vi "P4CMD Configure Project.vi"(8 "error in (no error)":errorcluster, 9 "configuration data in":string) -> (0 "error out":errorcluster, 1 "configuration data out":string, 2 "status message":string, 5 "dialog box cancelled?":bool)   [LabVIEW 2020, in "NI_SCC_P4CMD.lvlib"]
uses:
  <vilib>/SourceControl/Providers/P4CMD/NI_SCC_P4CMD.lvlib
  <vilib>/SourceControl/support/SCCSup Message Strings GLBL.vi
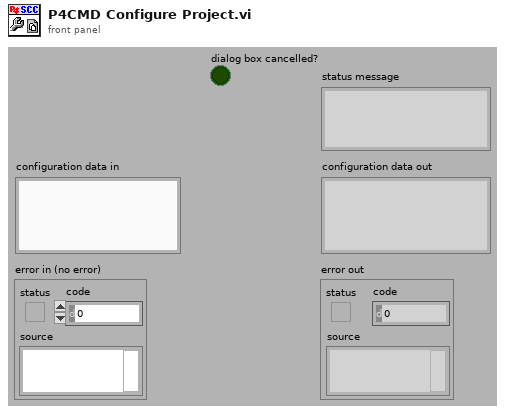
[diagram p1: front panel]
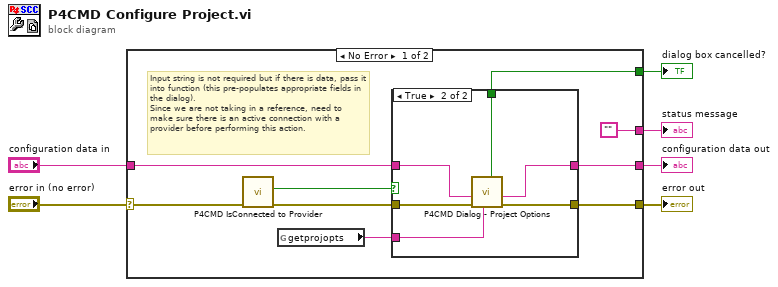
[diagram p0: block diagram]
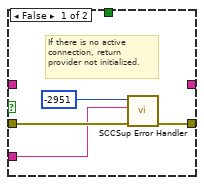
[diagram p2: hidden frame]
diagram:
  n1 = case shown="No Error" "error in (no error)" {
    selector: "error in (no error)" -> [w11 w26]
    tunnel: [w8 w26] -> w5
    tunnel: ["" _] -> w4
    tunnel: [w12 _] -> w3
    tunnel: [w13 _] -> w2
    tunnel: "configuration data in" -> [w14 _]
    frame No Error {
      # "Input string is not required but if there is data, pass it into function (this pre-populates appropriate fields in the dialog).\nSince we are not taking in a reference, need to make sure there is an active connection with a provider before performing this action."
      n2 = call <vilib>:"P4CMD IsConnected to Provider.vi"("error in (no error)"=w11) -> ("error out"=w10:errorcluster, "active connection?"=w9:bool)  [unwired: 9 in]
      n3 = global read "SCCSup Message Strings GLBL.vi" "getprojopts"() -> (w7:string)
      n4 = case shown="True" w9 {
        tunnel: w14 -> [_ w25]
        tunnel: [w18 w24] -> w8
        tunnel: [_ w23] -> w13
        tunnel: [_ w22] -> w12
        tunnel: w10 -> [w19 w21]
        tunnel: w7 -> [w16 w20]
        frame False {
          # "If there is no active connection, return provider not initialized."
          n5 = call <vilib>:"SCCSup Error Handler.vi"("error in (no error)"=w19, "operation message"=w16, "scc error code"=-2951 ("t")) -> ("error out"=w18:errorcluster)  [unwired: 8 in]
        }
        frame True {
          n6 = call <vilib>:"P4CMD Dialog - Project Options.vi"("operation message"=w20, "error in (no error)"=w21, "configuration data in"=w25) -> ("error out"=w24:errorcluster, "configuration data out"=w23:string, "cancelled?"=w22:bool)  [unwired: 6 in]
        }
      }
    }
    frame Error {
    }
  }
  "error out" <- w5
  "status message" <- w4
  "dialog box cancelled?" <- w3
  "configuration data out" <- w2
